vi "clk div.vi"(10 "divider":fxp<+,4,4>, 11 "enable divider":bool) -> (3 "f":bool)   [LabVIEW 2019]
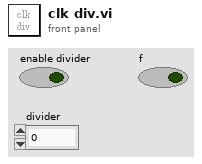
[diagram p1: front panel]
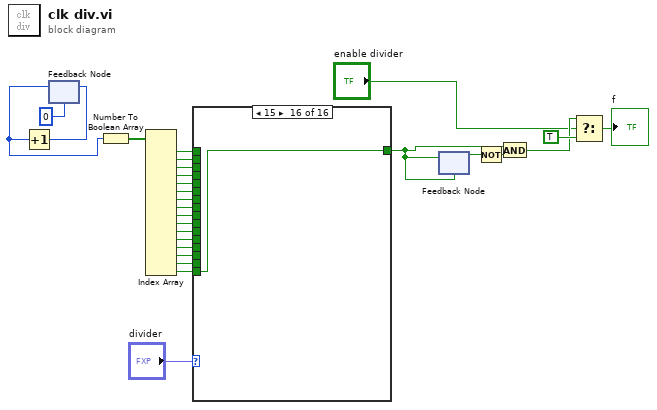
[diagram p0: block diagram]
diagram:
  n1 = feedback #1(u16 0) -> (w22:u16)
  n2 = Increment(x=w22) -> (x+1=w12:u16)
  n3 = feedback-in #1(w12) -> ()
  n4 = Number To Boolean Array(number=w22) -> (Boolean array=w10:bool[])
  n5 = Index Array(array=w10) -> (element #1=w13:bool, element #2=w14:bool, element #3=w15:bool, element #4=w16:bool, element #5=w17:bool, element #6=w18:bool, element #7=w19:bool, element #8=w20:bool, element #9=w8:bool, element #10=w7:bool, element #11=w6:bool, element #12=w5:bool, element #13=w4:bool, element #14=w3:bool, element #15=w2:bool, element #16=w1:bool)  [unwired: 16 in]
  n6 = case shown="15" "divider" {
    tunnel: w13 -> [w29 _ _ _ _ _ _ _ _ _ _ _ _ _ _ _]
    tunnel: w14 -> [_ w30 _ _ _ _ _ _ _ _ _ _ _ _ _ _]
    tunnel: w15 -> [_ _ w31 _ _ _ _ _ _ _ _ _ _ _ _ _]
    tunnel: w16 -> [_ _ _ w32 _ _ _ _ _ _ _ _ _ _ _ _]
    tunnel: w17 -> [_ _ _ _ w33 _ _ _ _ _ _ _ _ _ _ _]
    tunnel: w18 -> [_ _ _ _ _ w34 _ _ _ _ _ _ _ _ _ _]
    tunnel: w19 -> [_ _ _ _ _ _ w35 _ _ _ _ _ _ _ _ _]
    tunnel: w20 -> [_ _ _ _ _ _ _ w36 _ _ _ _ _ _ _ _]
    tunnel: [w29 w30 w31 w32 w33 w34 w35 w36 w37 w38 w39 w40 w41 w42 w43 w44] -> w24
    tunnel: w8 -> [_ _ _ _ _ _ _ _ w37 _ _ _ _ _ _ _]
    tunnel: w7 -> [_ _ _ _ _ _ _ _ _ w38 _ _ _ _ _ _]
    tunnel: w6 -> [_ _ _ _ _ _ _ _ _ _ w39 _ _ _ _ _]
    tunnel: w5 -> [_ _ _ _ _ _ _ _ _ _ _ w40 _ _ _ _]
    tunnel: w4 -> [_ _ _ _ _ _ _ _ _ _ _ _ w41 _ _ _]
    tunnel: w3 -> [_ _ _ _ _ _ _ _ _ _ _ _ _ w42 _ _]
    tunnel: w2 -> [_ _ _ _ _ _ _ _ _ _ _ _ _ _ w43 _]
    tunnel: w1 -> [_ _ _ _ _ _ _ _ _ _ _ _ _ _ _ w44]
    frame 0, Default {
    }
    frame 1 {
    }
    frame 2 {
    }
    frame 3 {
    }
    frame 4 {
    }
    frame 5 {
    }
    frame 6 {
    }
    frame 7 {
    }
    frame 8 {
    }
    frame 9 {
    }
    frame 10 {
    }
    frame 11 {
    }
    frame 12 {
    }
    frame 13 {
    }
    frame 14 {
    }
    frame 15 {
    }
  }
  n7 = feedback #2(w24) -> (w23:bool)
  n8 = feedback-in #2(w24) -> ()
  n9 = Not(x=w23) -> (.not. x?=w9:bool)
  n10 = And(x=w24, y=w9) -> (x .and. y?=w26:bool)
  n11 = Select(t=w26, s="enable divider", f=TRUE) -> (s? t:f=→"f":bool)
